vi "StateMachine (SubVI).vi"(9 "Activate":bool, 10 "Array":dbl[](array[numeric]), 11 "Step":u32) -> (2 "Numeric":dbl)   [LabVIEW 2012]
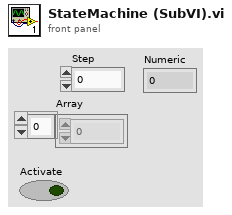
[diagram p1: front panel]
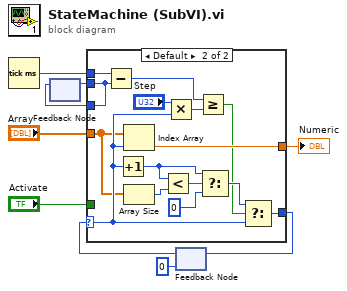
[diagram p0: block diagram]
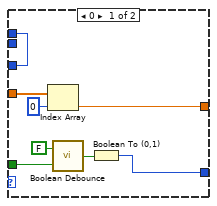
[diagram p2: hidden frame]
diagram:
  n1 = Tick Count (ms)() -> (millisecond timer value=w6:u32)
  n2 = feedback #1() -> (w7:u32)  [unwired: 1 in]
  n3 = feedback #2(0) -> (w3:i32)
  n4 = case shown="Default" w3 {
    selector: w3 -> [_ w29]
    tunnel: [w12 w32] -> w2
    tunnel: [w17 w30] -> w9
    tunnel: "Activate" -> [w11 _]
    tunnel: w6 -> [w14 w23]
    tunnel: w7 -> [_ w21]
    tunnel: [w14 w21] -> w8
    tunnel: "Array" -> [w13 w18]
    frame 0 {
      n5 = Index Array(array=w13, index=0) -> (element=w17:dbl)
      n6 = call "Boolean Debounce.vi"("Boolean in"=w11, "Default"=FALSE) -> ("Boolean out"=w10:bool)  [unwired: 1 in]
      n7 = Boolean To (0,1)(Boolean=w10) -> (0, 1=w12:i16)
    }
    frame Default {
      n8 = Subtract(x=w23, y=w21) -> (x-y=w22:u32)
      n9 = Increment(x=w29) -> (x+1=w24:i32)
      n10 = Index Array(array=w18, index=w29) -> (element=w30:dbl)
      n11 = Array Size(array=w18) -> (size(s)=w19:i32)
      n12 = Less?(x=w24, y=w19) -> (x < y?=w28:bool)
      n13 = Multiply(x="Step", y=w29) -> (x*y=w31:u32)
      n14 = Greater Or Equal?(x=w22, y=w31) -> (x >= y?=w25:bool)
      n15 = Select(t=w24, s=w28, f=0) -> (s? t:f=w26:i32)
      n16 = Select(t=w26, s=w25, f=w29) -> (s? t:f=w32:i32)
    }
  }
  "Numeric" <- w9
  n17 = feedback-in #1(w8) -> ()
  n18 = feedback-in #2(w2) -> ()
